vi "Script Name Msg.vi"(4 "Name":string, 6 "Name Msg":T1, 8 "error in":errorcluster) -> (0 "error out":errorcluster)   [LabVIEW 2020, in "_Rescript.lvlib" / "Msg.lvlib" / "Msg.lvclass"]
uses:
  Msg.lvclass
  _Rescript.lvlib
  Name Msg.ctl
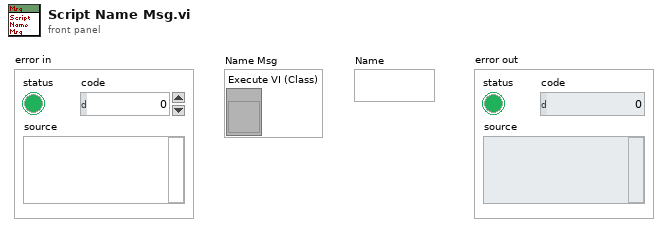
[diagram p1: front panel]
types:
  T1 = typedef "_Rescript.lvlib/Msg.lvlib/Msg.lvclass/Name Msg.ctl" = cluster{"Execute VI (Class)":refnum<vi>}
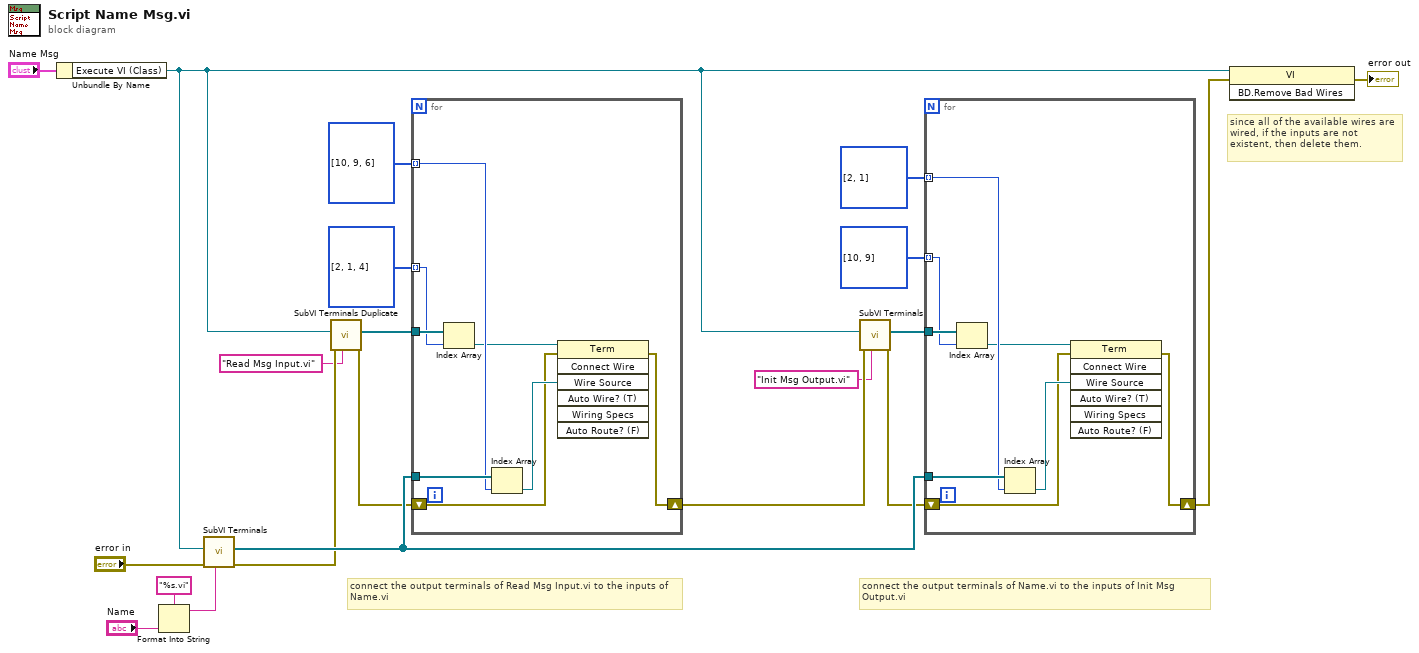
[diagram p0: block diagram]
diagram:
  # "since all of the available wires are wired, if the inputs are not existent, then delete them."
  # "connect the output terminals of Read Msg Input.vi to the inputs of Name.vi"
  # "connect the output terminals of Name.vi to the inputs of Init Msg Output.vi"
  n1 = Unbundle By Name("Name Msg") -> ("Execute VI (Class)"=w2:refnum<vi>)
  n2 = Format Into String(format string="%s.vi", "Name") -> (resulting string=w15:string)  [unwired: 2 in, 1 out]
  n3 = call "SubVI Terminals.vi"("Label"=w15, "error in"="error in", "VI"=w2) -> ("error out"=w5:errorcluster, "Terminals[]"=w16:refnum<vi>[])  [unwired: 7 in]
  n4 = call "SubVI Terminals Duplicate.vi"("Label"="Read Msg Input.vi", "error in"=w5, "VI"=w2) -> ("error out"=w4:errorcluster, "Terminals[]"=w1:refnum<vi>[])  [unwired: 7 in]
  n5 = for {
    tunnel: w1 -> [w29]
    tunnel: w16 -> [w28]
    tunnel: i32[] [2, 1, 4] ("Terminals Descending Order") -> [w27] mode=indexing
    tunnel: i32[] [10, 9, 6] ("Terminals Descending Order") -> [w26] mode=indexing
    shift-right: [w22] -> w11
    shift-left: w4 -> [w23]
    n6 = Index Array(array=w29, index=w27) -> (element=w25:refnum<vi>)
    n7 = Index Array(array=w28, index=w26) -> (element=w24:refnum<vi>)
    n8 = invoke class="Term" method="Connect Wire"(reference=w25, error in=w23, "Wire Source"=w24) -> (error out=w22:errorcluster)  [unwired: 4 in, 6 out]
  }
  n9 = call "SubVI Terminals.vi"("Label"="Init Msg Output.vi", "error in"=w11, "VI"=w2) -> ("error out"=w12:errorcluster, "Terminals[]"=w13:refnum<vi>[])  [unwired: 7 in]
  n10 = for {
    tunnel: w13 -> [w37]
    tunnel: w16 -> [w36]
    tunnel: i32[] [10, 9] ("Terminals Descending Order") -> [w35] mode=indexing
    tunnel: i32[] [2, 1] ("Terminals Descending Order") -> [w34] mode=indexing
    shift-right: [w30] -> w18
    shift-left: w12 -> [w31]
    n11 = Index Array(array=w37, index=w35) -> (element=w33:refnum<vi>)
    n12 = Index Array(array=w36, index=w34) -> (element=w32:refnum<vi>)
    n13 = invoke class="Term" method="Connect Wire"(reference=w33, error in=w31, "Wire Source"=w32) -> (error out=w30:errorcluster)  [unwired: 4 in, 6 out]
  }
  n14 = invoke class="VI" method="BD.Remove Bad Wires"(reference=w2, error in=w18) -> (error out=→"error out":errorcluster)  [unwired: 1 in, 2 out]
